vi "tearDown.vi"(8 "error in (no error)":errorcluster, 11 "reference in":refnum<class "testcase-CSMSyncMessage.lvclass">) -> (0 "error out":errorcluster, 3 "reference out":refnum<class "testcase-CSMSyncMessage.lvclass">)   [LabVIEW 2017, in "testcase-CSMSyncMessage.lvclass"]
doc: "tearDown runs after the test method has completed. Use this method to clean up any operations or references that were opened by setUp or the test method. Unit tests should be independent of other unit tests so this VI should ensure that the next test can run in a 'clean' test environment."
uses:
  testcase-CSMSyncMessage.lvclass
  testcase-CSMSyncMessage.lvclass/testcase-CSMSyncMessage.ctl
  src/user.lib/_NEVSTOP/Communicable State Machine(CSM)/Communicable State Machine.lvlib
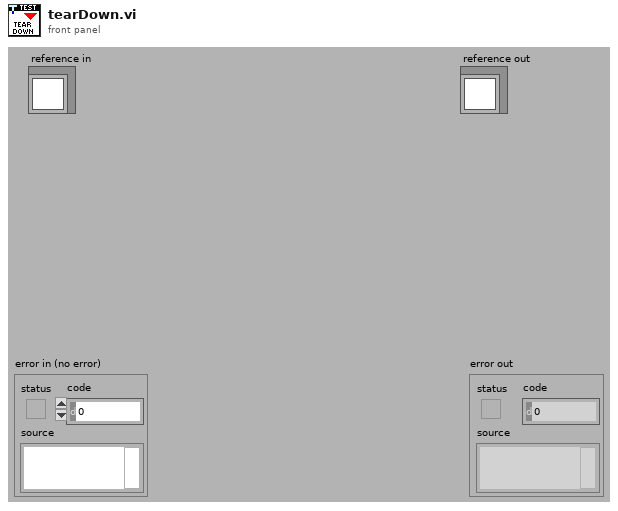
[diagram p1: front panel]
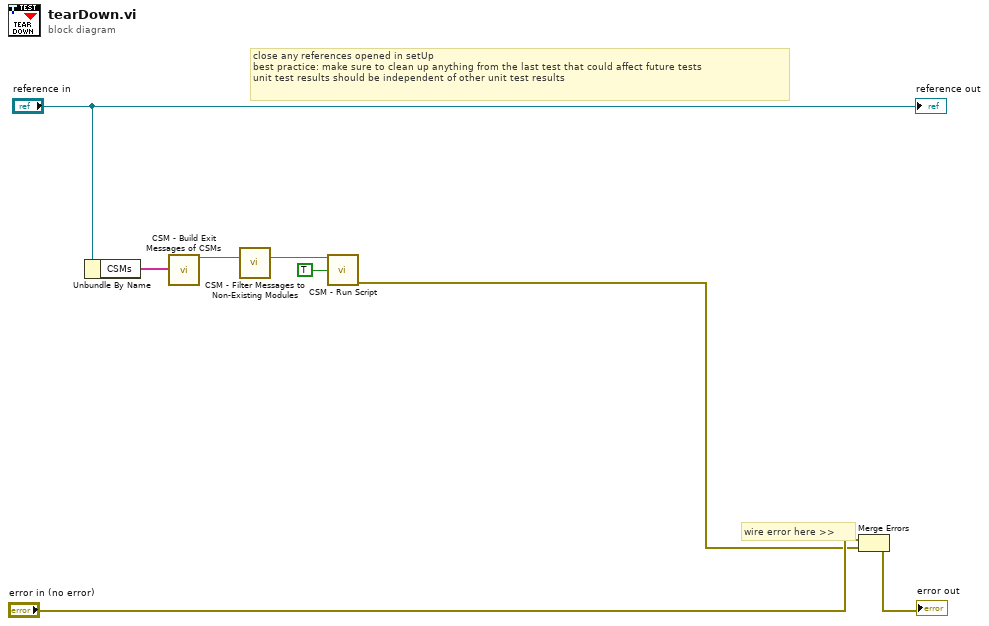
[diagram p0: block diagram]
diagram:
  # "wire error here >>"
  # "close any references opened in setUp\nbest practice: make sure to clean up anything from the last test that could affect future tests\nunit test results should be independent of other unit test results"
  n1 = Unbundle By Name("reference in") -> ("CSMs"=w5:string[])
  n2 = call "CSM - Build Exit Messages of CSMs.vi"("CSMs"=w5) -> ("States"=w4:string)  [unwired: 14 in]
  n3 = call "CSM - Filter Messages to Non-Existing Modules.vi"("State (S) In (\"\")"=w4) -> ("States Out"=w1:string)  [unwired: 14 in]
  n4 = call "CSM - Run Script.vi"("CSM Scripts"=w1, "Continue If Error? (F)"=TRUE) -> ("error out"=w2:errorcluster)  [unwired: 11 in, 2 out]
  n5 = Merge Errors("error in (no error)", w2) -> (→"error out":errorcluster)
  "reference out" <- "reference in"
